vi "ziExample-Module-DAQ_trigger.vi"() -> ()   [LabVIEW 2009]
doc: "Control a Zurich instrument device via the LabOne Labview API. \nRequirements: Zurich Instruments MFLI, HF2 or UHFLI \nThis example shows how to start a DAQ trigger module and retrieve the Data.\n\n© Zurich Instruments AG, www.zhinst.com"
uses:
  <instrlib>/Zurich Instruments LabOne/Public/Modules/ziTypeModEnum.ctl
  <instrlib>/Zurich Instruments LabOne/Public/Modules/ziModSetValueDouble.vi
  <instrlib>/Zurich Instruments LabOne/Public/Modules/ziModSetValueDoubleArray.vi
  <instrlib>/Zurich Instruments LabOne/Public/Modules/ziModSetValueBinaryArray.vi
  <instrlib>/Zurich Instruments LabOne/Public/Configure/ziSetValueDoubleArray.vi
  <instrlib>/Zurich Instruments LabOne/Public/Modules/ziModGetDoubleData.vi
  <instrlib>/Zurich Instruments LabOne/Zurich Instruments LabOne.lvlib
panel:
  in  "gridmode":bool
  out "Normal Demod X":dbl[][](graph)
  out "Grid DEMOD X":dbl[][](graph)
  out "Error Out":errorcluster
  in  "Address":string="DEV"
  out "Selected Device":string
  # "ziExample-Module-DAQ_trigger.vi\nRequirements: \n- HF2LI, UHFLI or MFLI \nsee block diagram for VI description"
  # "Tested Instruments:\n- HF2LI\n- UHFLI\n- MFLI"
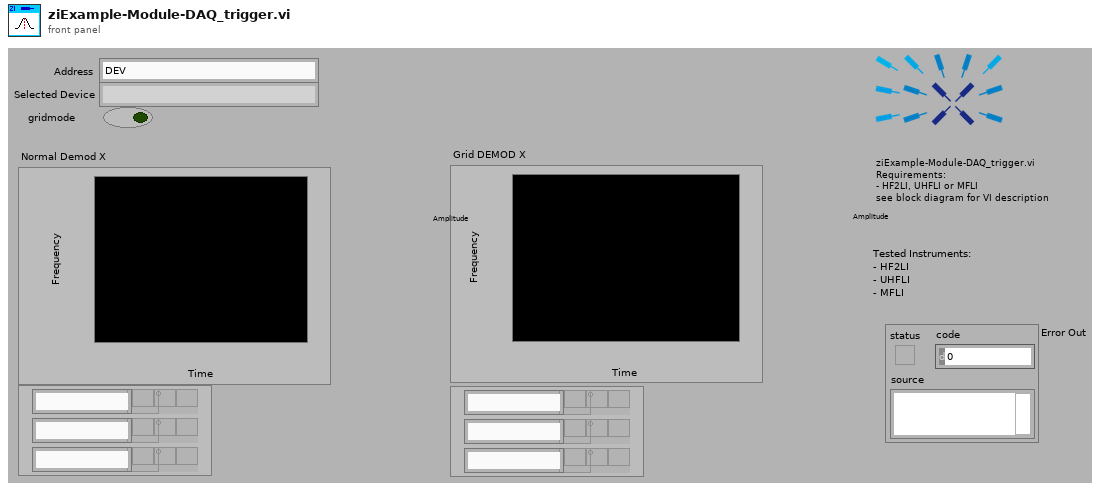
[diagram p1: front panel]
types:
  T1 = typedef "Zurich Instruments LabOne.lvlib/ziTypeModEnum.ctl" = u16
  T2 = typedef "Zurich Instruments LabOne.lvlib/ziTypeHandle.ctl" = cluster{"handleValid":bool, "Conn":u64, "Path Prefix":string, "Handle":u64, "Connected":bool, "Clockbase(s)":dbl}
  T3 = typedef "Zurich Instruments LabOne.lvlib/ziTypeModHandle.ctl" = cluster{"handleValid":bool, "Conn":u64, "ModHandle":u64, "moduleID":string, "Path Prefix":string}
  T4 = typedef "Zurich Instruments LabOne.lvlib/ziTypeModResults.ctl" = cluster{"PathArray":string[], "ValueType":T5, "NoOfResults":u64, "ziGenericHeader":T6[]}
  T5 = typedef "Zurich Instruments LabOne.lvlib/ziTypePollType.ctl" = enum16{"NONE", "DOUBLE_DATA", "INTEGER_DATA", "DEMOD_SAMPLE", "SCOPE_WAVE_HF2", "AUXIN_SAMPLE", "DIO_SAMPLE", "BYTE_ARRAY", "PWA_WAVE", "9", "10", "11", "12", "13", "14", "15", "TREE_CHANGE_DEPRI", "17", "ERROR", "19", "20", "21", "22", "23", "24", "25", "26", "27", "28", "29", "30", "31", "DOUBLE_DATA_TS", "INTEGER_DATA_TS", "34", "SCOPE_WAVE", "SCOPE_WAVE_EX", "37", "BYTE_ARRAY_TS", "39", "40", "41", "42", "43", "44", "45", "CNT_DATA", "47", "TREE_CHANGE", "49", "50", "51", "52", "53", "54", "55", "56", "57", "58", "59", "60", "61", "62", "63", "SWEEPER_DATA", "SPECTRUM_DATA", "ADVISOR_DATA", "VECTOR_DATA", "IMP_DATA"}
  T6 = typedef "Zurich Instruments LabOne.lvlib/ziTypeModGenericHeader.ctl" = cluster{"HeaderType":enum8{"HEADER_TYPE_NONE", "HEADER_TYPE_SWTRIGGER", "HEADER_TYPE_SWEEPER"}, "SampleFormat":u8, "SystemTime":timestamp, "CreatedTimeStamp":u64, "ChangedTimeStamp":u64, "Flags":u32, "ChunkSizeBytes":u64, "Name":string, "Status":u32, "GroupIndex":u32, "Color":u32, "ActiveRow":u32, "TriggerNumber":u64, "GridRows":u32, "GridCols":u32, "GridMode":u32, "GridOperation":u32, "GridDirection":u32, "GridRepetitions":u32, "GridColDelta":dbl, "GridColOffset":dbl, "GridRowDelta":dbl, "GridRowOffset":dbl, "Bandwidth":dbl, "Center":dbl, "Nenbw":dbl}
  T7 = typedef "Zurich Instruments LabOne.lvlib/ziTypeDoubleDataTSGrid.ctl" = cluster{"Timestamp (ticks)":u64[][], "Value":dbl[][]}
  T8 = typedef "Zurich Instruments LabOne.lvlib/ziTypeDoubleDataTS.ctl" = cluster{"Timestamp (ticks)":u64[], "Value":dbl[]}
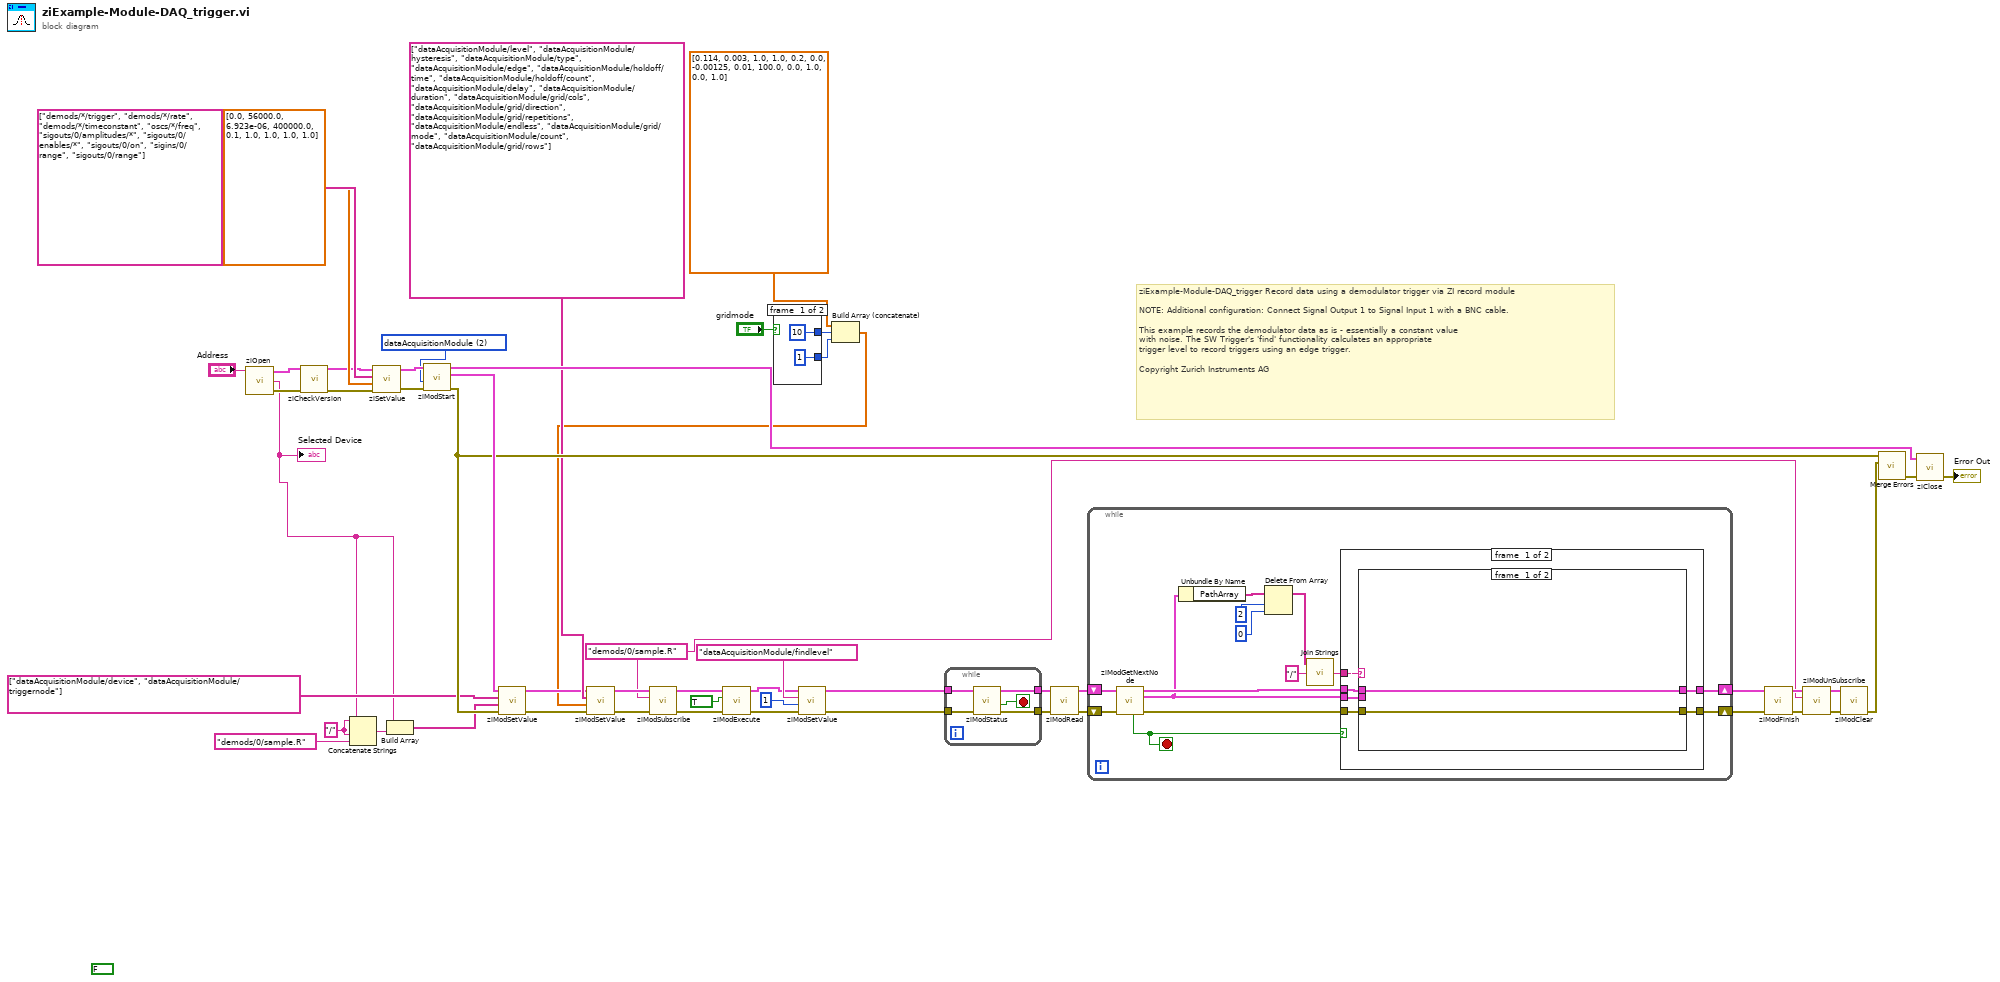
[diagram p0: block diagram]
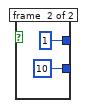
[diagram p2: hidden frame]
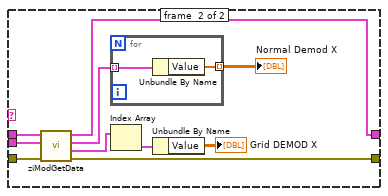
[diagram p3: hidden frame]
diagram:
  w1 = T1 2 items=["sweep", "scopeModule", "dataAcquisitionModule", "pidAdvisor", "awgModule", "impedanceModule", "multiDeviceSyncModule", "zoomFFT", "trigger", "deviceSettings", "record"] ("module Id")
  w10 = "/"
  w8 = "demods/0/sample.R" ("subscribe")
  (unwired) FALSE ("stop")
  # "ziExample-Module-DAQ_trigger Record data using a demodulator trigger via ZI record module\n \nNOTE: Additional configuration: Connect Signal Output 1 to Signal Input 1 with a BNC cable.\n\nThis example records the demodulator data as is - essentially a constant value\nwith noise. The SW Trigger's 'find' functionality calculates an appropriate\ntrigger level to record triggers using an edge trigger.\n\nCopyright Zurich Instruments AG"
  n1 = call <instrlib>:"ziOpen.vi"("Address"="Address") -> ("Error Out"=w36:errorcluster, "Selected Device"=w9:string, "HandleOut"=w39:T2)  [unwired: 1 in, 2 out]
  "Selected Device" <- w9
  n2 = call <instrlib>:"ziCheckVersion.vi"("Handle In"=w39, "Error In"=w36) -> ("Handle Out"=w38:T2, "Error Out"=w37:errorcluster)  [unwired: 11 in, 1 out]
  n3 = Concatenate Strings(w10, w9, w10, "demods/0/sample.R" ("element")) -> (w7:string)
  n4 = call-poly <instrlib>:"ziSetValue.vi"("Error In"=w37, "Values"=dbl[] [0.0, 56000.0, 6.923e-06, 400000.0, 0.1, 1.0, 1.0, 1.0, 1.0], "Paths"=string[] ["demods/*/trigger", "demods/*/rate", "demods/*/timeconstant", "oscs/*/freq", "sigouts/0/amplitudes/*", "sigouts/0/enables/*", "sigouts/0/on", "sigins/0/range", "sigouts/0/range"], "Handle In"=w38) -> ("Error Out"=w46:errorcluster, "Handle Out"=w45:T2)  [unwired: 1 in]
  n5 = Build Array(w9, w7) -> (w29:string[])
  n6 = call <instrlib>:"ziModStart.vi"("Error In"=w46, "module Id"=w1, "Handle In"=w45) -> ("Error Out"=w41:errorcluster, "ModHandle Out"=w44:T3, "Handle Out"=w40:T2)  [unwired: 6 in]
  n7 = call-poly <instrlib>:"ziModSetValue.vi"("Error In"=w41, "Values"=w29, "Paths"=string[] ["dataAcquisitionModule/device", "dataAcquisitionModule/triggernode"], "ModHandle In"=w44) -> ("Error Out"=w26:errorcluster, "ModHandle Out"=w27:T3)  [unwired: 6 in]
  n8 = case shown="False" "gridmode" {
    tunnel: [10 1] -> w4
    tunnel: [1 10] -> w3
    frame #0 {
    }
    frame #1 {
    }
  }
  n9 = Build Array (concatenate)(dbl[] [0.114, 0.003, 1.0, 1.0, 0.2, 0.0, -0.00125, 0.01, 100.0, 0.0, 1.0, 0.0, 1.0], w4, w3) -> (w2:dbl[])
  n10 = call-poly <instrlib>:"ziModSetValue.vi"("Error In"=w26, "Values"=w2, "Paths"=string[] ["dataAcquisitionModule/level", "dataAcquisitionModule/hysteresis", "dataAcquisitionModule/type", "dataAcquisitionModule/edge", "dataAcquisitionModule/holdoff/time", "dataAcquisitionModule/holdoff/count", "dataAcquisitionModule/delay", "dataAcquisitionModule/duration", "dataAcquisitionModule/grid/cols", "dataAcquisitionModule/grid/direction", "dataAcquisitionModule/grid/repetitions", "dataAcquisitionModule/endless", "dataAcquisitionModule/grid/mode", "dataAcquisitionModule/count", "dataAcquisitionModule/grid/rows"], "ModHandle In"=w27) -> ("Error Out"=w20:errorcluster, "ModHandle Out"=w21:T3)  [unwired: 6 in]
  n11 = call <instrlib>:"ziModSubscribe.vi"("Error In"=w20, "Path"=w8, "ModHandle In"=w21) -> ("Error Out"=w24:errorcluster, "ModHandle Out"=w25:T3)  [unwired: 6 in]
  n12 = call <instrlib>:"ziModExecute.vi"("Error In"=w24, "Modal (F)"=TRUE, "ziModHandle In"=w25) -> ("Error Out"=w16:errorcluster, "ziModHandle Out"=w19:T3)  [unwired: 5 in, 1 out]
  n13 = call-poly <instrlib>:"ziModSetValue.vi"("Error In"=w16, "Value"=1, "Path"="dataAcquisitionModule/findlevel", "ModHandle In"=w19) -> ("Error Out"=w17:errorcluster, "ModHandle Out"=w18:T3)  [unwired: 6 in]
  n14 = while {
    tunnel: w18 -> [w61]
    tunnel: w17 -> [w60]
    tunnel: [w58] -> w13
    tunnel: [w57] -> w12
    stop <- w59 stop-if-true
    n15 = call <instrlib>:"ziModStatus.vi"("Error In"=w60, "ModHandle IN"=w61) -> ("Error Out"=w57:errorcluster, "Finished?"=w59:bool, "ModHandle Out"=w58:T3)  [unwired: 5 in, 1 out]
  }
  n16 = call <instrlib>:"ziModRead.vi"("error in"=w12, "ziModHandle In"=w13) -> ("error out"=w15:errorcluster, "ziModHandle Out"=w14:T3)  [unwired: 8 in]
  n17 = while {
    shift-right: [w70] -> w32
    shift-left: w14 -> [w74]
    shift-right: [w71] -> w33
    shift-left: w15 -> [w75]
    stop <- w69 stop-if-true
    n18 = call <instrlib>:"ziModGetNextNode.vi"("Error In"=w75, "ModHandle In"=w74) -> ("Error Out"=w72:errorcluster, "ModResults"=w68:T4, "ModHandle Out"=w73:T3, "NoData"=w69:bool)  [unwired: 6 in]
    n19 = Unbundle By Name(w68) -> ("PathArray"=w67:string[])
    n20 = Delete From Array(array=w67, length=2, index=0) -> (array with subset deleted=w64:string[])  [unwired: 1 out]
    n21 = call <vilib>:"Join Strings.vi"("Separator (,)"="/", "Strings In"=w64) -> ("String"=w62:string)  [unwired: 1 in]
    n22 = case shown="False" w69 {
      tunnel: w68 -> [w81 _]
      tunnel: w73 -> [w80 w97]
      tunnel: w72 -> [w79 w96]
      tunnel: [w78 w96] -> w71
      tunnel: [w77 w97] -> w70
      tunnel: w62 -> [w76 _]
      frame #0 {
        n23 = case shown="\"demods/0/sample.R\"" w76 {
          tunnel: w80 -> [w83 w87]
          tunnel: w81 -> [_ w86]
          tunnel: w79 -> [w82 w90]
          tunnel: [w82 w92] -> w78
          tunnel: [w83 w93] -> w77
          frame #0 {
          }
          frame #1 {
            n24 = call-poly <instrlib>:"ziModGetData.vi"("Error In"=w90, "ModResults"=w86, "ModHandle In"=w87) -> ("Error Out"=w92:errorcluster, "DoubleSampleGrid"=w89:T7[], "DoubleSample"=w91:T8[], "ModHandle Out"=w93:T3)  [unwired: 4 in, 1 out]
            n25 = for {
              tunnel: w91 -> [w95] mode=indexing
              tunnel: [w94] -> w84 mode=indexing
              n26 = Unbundle By Name(w95) -> ("Value"=w94:dbl[])
            }
            "Normal Demod X" <- w84
            n27 = Index Array(array=w89) -> (element=w88:T7)  [unwired: 1 in]
            n28 = Unbundle By Name(w88) -> ("Value"=→"Grid DEMOD X":dbl[][])
          }
        }
      }
      frame #1 {
      }
    }
  }
  n29 = call <instrlib>:"ziModFinish.vi"("Error In"=w33, "ziModHandle In"=w32) -> ("Error Out"=w34:errorcluster, "ziModHandle Out"=w31:T3)  [unwired: 7 in]
  n30 = call <instrlib>:"ziModUnSubscribe.vi"("Error In"=w34, "Path (\"/\")"=w8, "ModHandle In"=w31) -> ("Error Out"=w51:errorcluster, "ModHandle Out"=w50:T3)  [unwired: 7 in]
  n31 = call <instrlib>:"ziModClear.vi"("Error In"=w51, "ziModHandle In"=w50) -> ("Error Out"=w43:errorcluster)  [unwired: 7 in, 1 out]
  n32 = call <vilib>:"Merge Errors.vi"("error in 2 (no error)"=w43, "error in 1 (no error)"=w41) -> ("error out"=w42:errorcluster)  [unwired: 5 in]
  n33 = call <instrlib>:"ziClose.vi"("Error In"=w42, "Handle In"=w40) -> ("Error Out"=→"Error Out":errorcluster)  [unwired: 2 in, 1 out]
